vi "CRYGet Visa Information.vi"(8 "error in":errorcluster, 11 "Hardware":string) -> (0 "error out":errorcluster)   [LabVIEW 2013]
uses:
  Program/CRYRef nums global.vi
panel:
  in  "VISA serial ports (empty array)":T1(array[cluster]) {"COM port (1 = COM1, etc.)" min=1 max=99}
  in  "VISA session (for class)":refnum<visa-resource-name>
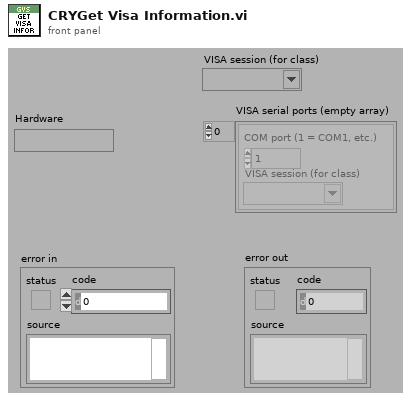
[diagram p1: front panel]
types:
  T1 = cluster{"COM port (1 = COM1, etc.)":i32, "VISA session (for class)":refnum<visa-resource-name>}[]
  T2 = typedef "CRYHardware.ctl" = cluster{"Name":string, "Analog I/O":u16, "Digital I/O":u16, "Channels":u8, "Dig Dev ID":u8, "N ports":u8, "Interface":u32, "Dig I/O Ports":cluster{"port #":i16, "width":i16, "direction":i32}[], "Interf settings":cluster{"Type":u16, "COM Port":u8, "Baud rate":u32, "Data bits":u32, "Parity":u16, "Stop bits":u16, "Flow control":u16, "Dev ID IEEE":u8}[], "N interfs":i32, "udev SNs":i16[], "udev enable":bool, "Channel Array":T3[], "Cal sequence":string, "SelectedIn":u16, "SelectedOut":u16, "SelectedTab":u16, "State":bool, "Help":string, "Advanced":bool, "In Audio Driver":u16, "Out Audio Driver":u16}
  T3 = typedef "CRYHardware Channel Info.ctl" = cluster{"ID":i32, "Name":string, "Digital":bool, "Input":bool, "Device Name":string, "Hardware Ch ID":u8, "Vmax (V)":dbl, "Latency (samples)":dbl, "Sampling Rate (Hz)":u32, "Bit Depth":u32, "Anti-aliasing Factor (%fs)":sgl, "DAQmx Channel":tag, "term config":i32, "Coupling":i32, "IEPE en":bool, "ASIOChannel Name":string, "Audio Driver":u16, "ASIOChannel Index":u8}
  T4 = cluster{"Type":u16, "COM Port":u8, "Baud rate":u32, "Data bits":u32, "Parity":u16, "Stop bits":u16, "Flow control":u16, "Dev ID IEEE":u8}[]
  T5 = cluster{"input XON/XOFF":bool, "input HW Handshake":bool, "input alt HW HShk":bool, "output XON/XOFF":bool, "output HW Handshake":bool, "output alt HW HShk":bool, "XOFF byte":u8, "XON byte":u8, "parity error byte":u16}
  T6 = cluster{i32, "VISA session (for class)":refnum<visa-resource-name>}
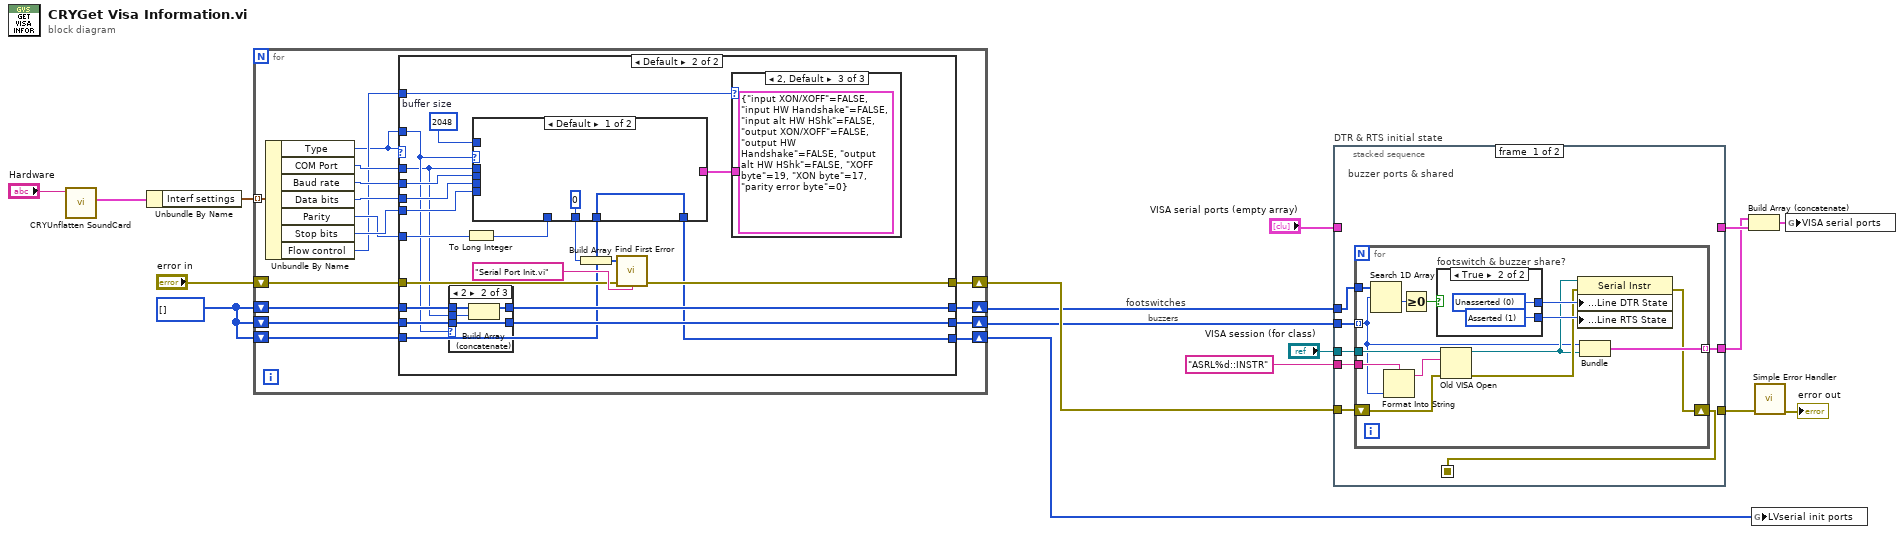
[diagram p0: block diagram]
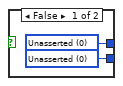
[diagram p2: hidden frame]
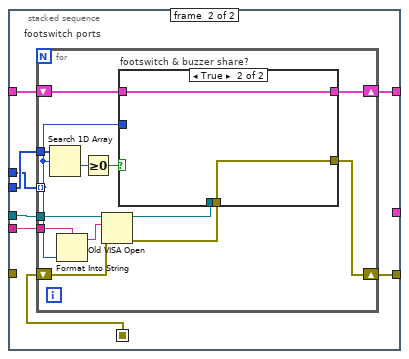
[diagram p3: hidden frame]
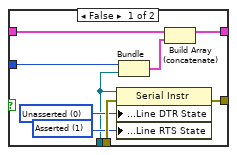
[diagram p4: hidden frame]
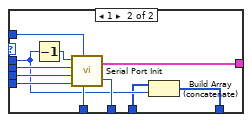
[diagram p6: hidden frame]
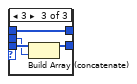
[diagram p8: hidden frame]
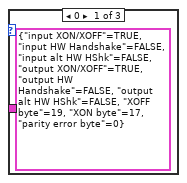
[diagram p9: hidden frame]
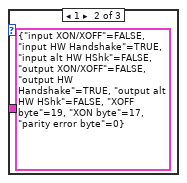
[diagram p10: hidden frame]
diagram:
  w17 = i32[] []
  # "buzzers"
  # "footswitches"
  n1 = call "CRYUnflatten SoundCard.vi"("Flatten SoundCard"="Hardware") -> ("SoundCard"=w2:T2)  [unwired: 8 in, 2 out]
  n2 = Unbundle By Name(w2) -> ("Interf settings"=w16:T4)
  n3 = for {
    shift-right: [w32] -> w10
    shift-left: "error in" -> [w33]
    tunnel: w16 -> [w31] mode=indexing
    shift-right: [w21] -> w9
    shift-left: w17 -> [w24]
    shift-right: [w20] -> w8
    shift-left: w17 -> [w23]
    shift-right: [w18] -> w6
    shift-left: w17 -> [w19]
    n4 = Unbundle By Name(w31) -> ("Type"=w22:u16, "COM Port"=w30:u8, "Baud rate"=w29:u32, "Data bits"=w28:u32, "Parity"=w26:u16, "Stop bits"=w27:u16, "Flow control"=w25:u16)
    n5 = case shown="Default" w22 {
      tunnel: w33 -> [w37 w54]
      tunnel: [w37 w53] -> w32
      tunnel: w30 -> [_ w40]
      tunnel: w29 -> [_ w52]
      tunnel: w28 -> [_ w51]
      tunnel: w27 -> [_ w50]
      tunnel: w26 -> [_ w49]
      tunnel: w25 -> [_ w48]
      tunnel: w24 -> [w36 w47]
      tunnel: w23 -> [w35 w46]
      tunnel: w22 -> [_ w42]
      tunnel: [w36 w45] -> w21
      tunnel: [w35 w44] -> w20
      tunnel: w19 -> [w34 w39]
      tunnel: [w34 w38] -> w18
      frame 0 {
      }
      frame Default {
        w41 = u16 2048  # buffer size
        n6 = case shown="2" w42 {
          tunnel: [w73 w75 w81] -> w45
          tunnel: w47 -> [w73 w76 w81]
          tunnel: [w72 w77 w78] -> w44
          tunnel: w46 -> [w72 w77 w80]
          tunnel: w40 -> [_ w74 w79]
          frame Default {
          }
          frame 2 {
            n7 = Build Array (concatenate)(w76, w74) -> (w75:i32[])
          }
          frame 3 {
            n8 = Build Array (concatenate)(w80, w79) -> (w78:i32[])
          }
        }
        n9 = To Long Integer(number=w49) -> (32bit integer=w55:i32)
        n10 = case shown="2, Default" w48 {
          tunnel: [T5 {"input XON/XOFF"=TRUE, "input HW Handshake"=FALSE, "input alt HW HShk"=FALSE, "output XON/XOFF"=TRUE, "output HW Handshake"=FALSE, "output alt HW HShk"=FALSE, "XOFF byte"=19, "XON byte"=17, "parity error byte"=0} ("flow control etc.") T5 {"input XON/XOFF"=FALSE, "input HW Handshake"=TRUE, "input alt HW HShk"=FALSE, "output XON/XOFF"=FALSE, "output HW Handshake"=TRUE, "output alt HW HShk"=FALSE, "XOFF byte"=19, "XON byte"=17, "parity error byte"=0} ("flow control etc.") T5 {"input XON/XOFF"=FALSE, "input HW Handshake"=FALSE, "input alt HW HShk"=FALSE, "output XON/XOFF"=FALSE, "output HW Handshake"=FALSE, "output alt HW HShk"=FALSE, "XOFF byte"=19, "XON byte"=17, "parity error byte"=0} ("flow control etc.")] -> w58
          frame 0 {
          }
          frame 1 {
          }
          frame 2, Default {
          }
        }
        n11 = case shown="Default" w42 {
          tunnel: w58 -> [_ w71]
          tunnel: w55 -> [_ w70]
          tunnel: w52 -> [_ w69]
          tunnel: w51 -> [_ w68]
          tunnel: w50 -> [_ w67]
          tunnel: [0 ("error code") w66] -> w43
          tunnel: w40 -> [_ w63]
          tunnel: w41 -> [_ w65]
          tunnel: w39 -> [w59 w62]
          tunnel: [w59 w61] -> w38
          frame Default {
          }
          frame 1 {
            n12 = Decrement(x=w63) -> (x-1=w64:u8)
            n13 = call <vilib>:"Serial Port Init.vi"("flow control etc."=w71, "parity"=w70, "buffer size"=w65, "stop bits"=w67, "data bits"=w68, "baud rate"=w69, "port number"=w64) -> ("error code"=w66:i32)
            n14 = Build Array (concatenate)(w62, w63) -> (w61:i32[])
          }
        }
        n15 = Build Array(w43) -> (w57:i32[])
        n16 = call <vilib>:"Find First Error.vi"("error in (no error)"=w54, "source messages"="Serial Port Init.vi", "error codes"=w57) -> ("error out"=w53:errorcluster)  [unwired: 1 in, 1 out]
      }
    }
  }
  n17 = stacked-sequence "DTR & RTS initial state" {
    seq-local: [w86 _] -> [_ w115]
    tunnel: w8 -> [w91 w117]
    tunnel: w9 -> [w90 w116]
    tunnel: "VISA session (for class)" -> [w89 w113]
    tunnel: "ASRL%d::INSTR" -> [w88 w112]
    tunnel: w10 -> [w87 _]
    tunnel: [w85 _] -> w12
    tunnel: [_ w114] -> w11
    tunnel: "VISA serial ports (empty array)" -> [_ w111]
    tunnel: [_ w110] -> w13
    frame #0 {
      # "buzzer ports & shared"
      n18 = for {
        tunnel: w91 -> [w95] mode=indexing
        tunnel: w90 -> [w105]
        tunnel: w89 -> [w101]
        tunnel: w88 -> [w100]
        tunnel: [w94] -> w85 mode=indexing
        shift-right: [w92] -> w86
        shift-left: w87 -> [w93]
        n19 = Search 1D Array(1D array=w105, element=w95) -> (index of element=w104:i32)  [unwired: 1 in]
        n20 = Format Into String(format string=w100, w95) -> (resulting string=w102:string)  [unwired: 2 in, 1 out]
        n21 = Greater Or Equal To 0?(x=w104) -> (x >= 0?=w103:bool)
        n22 = case "footswitch & buzzer share?" shown="True" w103 {
          tunnel: [w107 w109] -> w99
          tunnel: [w106 w108] -> w98
          frame False {
            w107 = i16 0 items=["Unknown"=-1, "Unasserted"=0, "Asserted"=1] ("Modem Line Settings:Line DTR State")
            w106 = i16 0 items=["Unknown"=-1, "Unasserted"=0, "Asserted"=1] ("Modem Line Settings:Line RTS State")
          }
          frame True {
            w109 = i16 0 items=["Unknown"=-1, "Unasserted"=0, "Asserted"=1] ("Modem Line Settings:Line DTR State")
            w108 = i16 1 items=["Unknown"=-1, "Unasserted"=0, "Asserted"=1] ("Modem Line Settings:Line RTS State")
          }
        }
        n23 = Old VISA Open(8:w93, 10:w102, 11:w101) -> (0:w97:errorcluster, 3:w96:refnum<visa-resource-name>)  [unwired: 2 in]
        n24 = property class="Serial Instr"(reference=w96, error in=w97, "Serial Settings:Modem Line Settings:Line DTR State"=w99, "Serial Settings:Modem Line Settings:Line RTS State"=w98) -> (error out=w92:errorcluster)  [unwired: 1 out]
        n25 = Bundle(w95, "VISA session (for class)"=w96) -> (w94:T6)  [unwired: 1 in]
      }
    }
    frame #1 {
      # "footswitch ports"
      n26 = for {
        tunnel: w116 -> [w120] mode=indexing
        tunnel: w117 -> [w130]
        tunnel: w113 -> [w126]
        tunnel: w112 -> [w125]
        shift-right: [w121] -> w114
        shift-left: w115 -> [w124]
        shift-right: [w118] -> w110
        shift-left: w111 -> [w119]
        n27 = Search 1D Array(1D array=w130, element=w120) -> (index of element=w129:i32)  [unwired: 1 in]
        n28 = Format Into String(format string=w125, w120) -> (resulting string=w127:string)  [unwired: 2 in, 1 out]
        n29 = Greater Or Equal To 0?(x=w129) -> (x >= 0?=w128:bool)
        n30 = Old VISA Open(8:w124, 10:w127, 11:w126) -> (0:w122:errorcluster, 3:w123:refnum<visa-resource-name>)  [unwired: 2 in]
        n31 = case "footswitch & buzzer share?" shown="True" w128 {
          tunnel: w123 -> [w134 _]
          tunnel: w122 -> [w139 w141]
          tunnel: [w136 w141] -> w121
          tunnel: w120 -> [w135 _]
          tunnel: w119 -> [w133 w140]
          tunnel: [w132 w140] -> w118
          frame False {
            w138 = i16 0 items=["Unknown"=-1, "Unasserted"=0, "Asserted"=1] ("Modem Line Settings:Line DTR State")
            w137 = i16 1 items=["Unknown"=-1, "Unasserted"=0, "Asserted"=1] ("Modem Line Settings:Line RTS State")
            n32 = property class="Serial Instr"(reference=w134, error in=w139, "Serial Settings:Modem Line Settings:Line DTR State"=w138, "Serial Settings:Modem Line Settings:Line RTS State"=w137) -> (error out=w136:errorcluster)  [unwired: 1 out]
            n33 = Bundle(w135, "VISA session (for class)"=w134) -> (w131:T6)  [unwired: 1 in]
            n34 = Build Array (concatenate)(w133, w131) -> (w132:T1)
          }
          frame True {
          }
        }
      }
    }
  }
  n35 = Build Array (concatenate)(w12, w13) -> (w7:T1)
  n36 = global write "CRYRef nums global.vi" "LVserial init ports"(w6) -> ()
  n37 = call <vilib>:"Simple Error Handler.vi"("error in (no error)"=w11) -> ("error out"=→"error out":errorcluster)  [unwired: 4 in, 4 out]
  n38 = global write "CRYRef nums global.vi" "VISA serial ports"(w7) -> ()
